vi "Configure Limit Function.vi"(7 "Upper Limit (1)":dbl=1.0 format="%.3f", 8 "error in (no error)":errorcluster, 9 "Enable Limit Operation (T:Enable)":bool=TRUE, 10 "Lower Limit (-1)":dbl=-1.0 format="%.3f", 11 "VISA resource name":refnum<visa-resource-name>) -> (0 "error out":errorcluster, 3 "VISA resource name out":refnum<visa-resource-name>="1")   [LabVIEW 2020, in "BK Precision 5491B.lvlib"]
doc: "Configures and enables the limit operation.\n\n<b>Note: Limit operation applies to the primary measurement function only.</b>"
uses:
  <instrlib>/BK Precision 5491B/BK Precision 5491B.lvlib
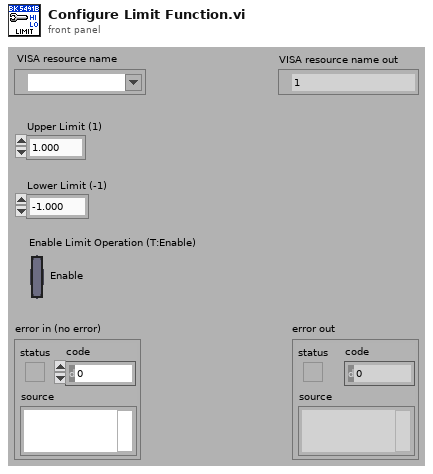
[diagram p1: front panel]
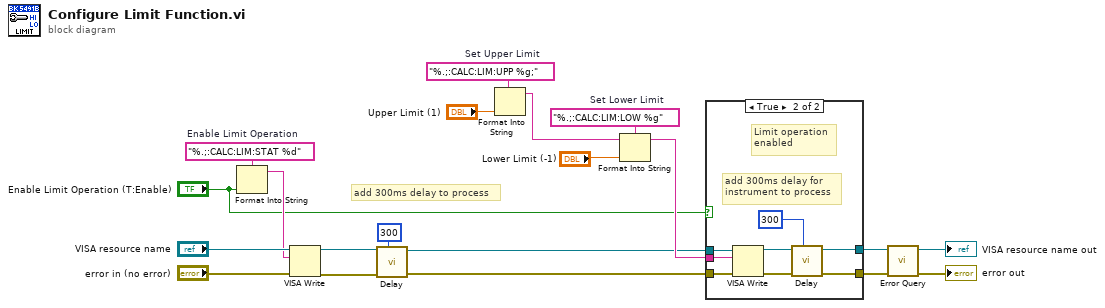
[diagram p0: block diagram]
diagram:
  w12 = "%.;:CALC:LIM:LOW %g"  # Set Lower Limit
  w14 = "%.;:CALC:LIM:STAT %d"  # Enable Limit Operation
  w18 = "%.;:CALC:LIM:UPP %g;"  # Set Upper Limit
  # "add 300ms delay to process"
  n1 = Format Into String(format string=w14, "Enable Limit Operation (T:Enable)") -> (resulting string=w8:string)  [unwired: 2 in, 1 out]
  n2 = VISA Write(VISA resource name="VISA resource name", write buffer=w8, error in (no error)="error in (no error)") -> (VISA resource name out=w6:refnum<visa-resource-name>, error out=w5:errorcluster)  [unwired: 1 out]
  n3 = call <instrlib>:"Delay.vi"("Delay Time (0)"=u32 300, "error in (no error)"=w5, "VISA resource name"=w6) -> ("error out"=w2:errorcluster, "VISA resource name out"=w3:refnum<visa-resource-name>)  [unwired: 7 in]
  n4 = Format Into String(format string=w18, "Upper Limit (1)") -> (resulting string=w11:string)  [unwired: 2 in, 1 out]
  n5 = Format Into String(format string=w12, initial string=w11, "Lower Limit (-1)") -> (resulting string=w7:string)  [unwired: 1 in, 1 out]
  n6 = case shown="True" "Enable Limit Operation (T:Enable)" {
    tunnel: [w22 w29] -> w17
    tunnel: [w21 w28] -> w16
    tunnel: w7 -> [_ w25]
    tunnel: w3 -> [w22 w24]
    tunnel: w2 -> [w21 w23]
    frame False {
      # "Limit operation\ndisabled"
    }
    frame True {
      # "Limit operation\nenabled"
      # "add 300ms delay for\ninstrument to process"
      n7 = VISA Write(VISA resource name=w24, write buffer=w25, error in (no error)=w23) -> (VISA resource name out=w30:refnum<visa-resource-name>, error out=w27:errorcluster)  [unwired: 1 out]
      n8 = call <instrlib>:"Delay.vi"("Delay Time (0)"=u32 300, "error in (no error)"=w27, "VISA resource name"=w30) -> ("error out"=w28:errorcluster, "VISA resource name out"=w29:refnum<visa-resource-name>)  [unwired: 7 in]
    }
  }
  n9 = call <instrlib>:"Error Query.vi"("error in (no error)"=w16, "VISA resource name"=w17) -> ("error out"=→"error out":errorcluster, "VISA resource name out"=→"VISA resource name out":refnum<visa-resource-name>)  [unwired: 7 in, 1 out]
